vi "PeelDataCheck.vi"() -> ()   [LabVIEW 2012]
uses:
  <vilib>/addons/database/Connection.llb/DB Tools Open Connec (Path).vi
  <vilib>/addons/database/Connection.llb/Conn Execute.vi
  <vilib>/addons/database/Recordset.llb/Rec Fetch Recordset Data (R).vi
  <vilib>/addons/database/Recordset.llb/Rec Destroy - Connection.vi
  <vilib>/addons/database/_DB Variant To Data/Database Variant To Data.xnode
  <vilib>/addons/database/NI_Database_API.lvlib
  <vilib>/Utility/SMTP/NI_SMTPEmail.lvlib
panel:
  out "spreadsheet string":string
  out "array":string[][](array[string])
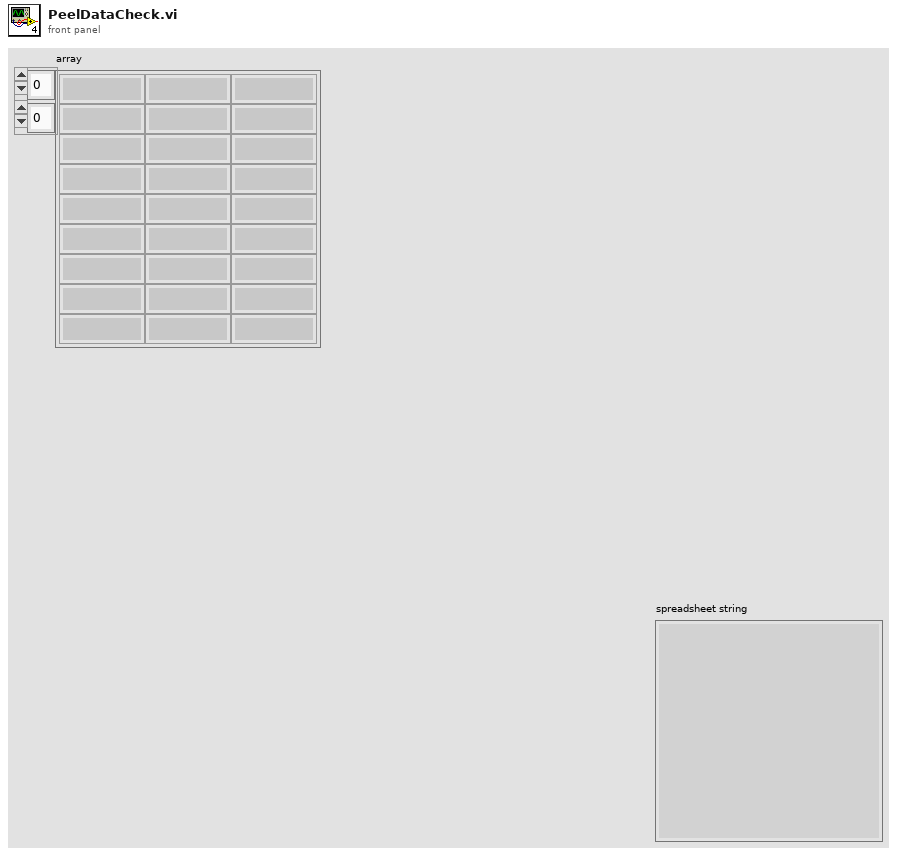
[diagram p1: front panel]
types:
  T1 = typedef "NI_Database_API.lvlib/Conn ObjectReference.ctl" = refnum<k1>
  T2 = typedef "NI_Database_API.lvlib/Rec ObjectReference.ctl" = refnum<k1>
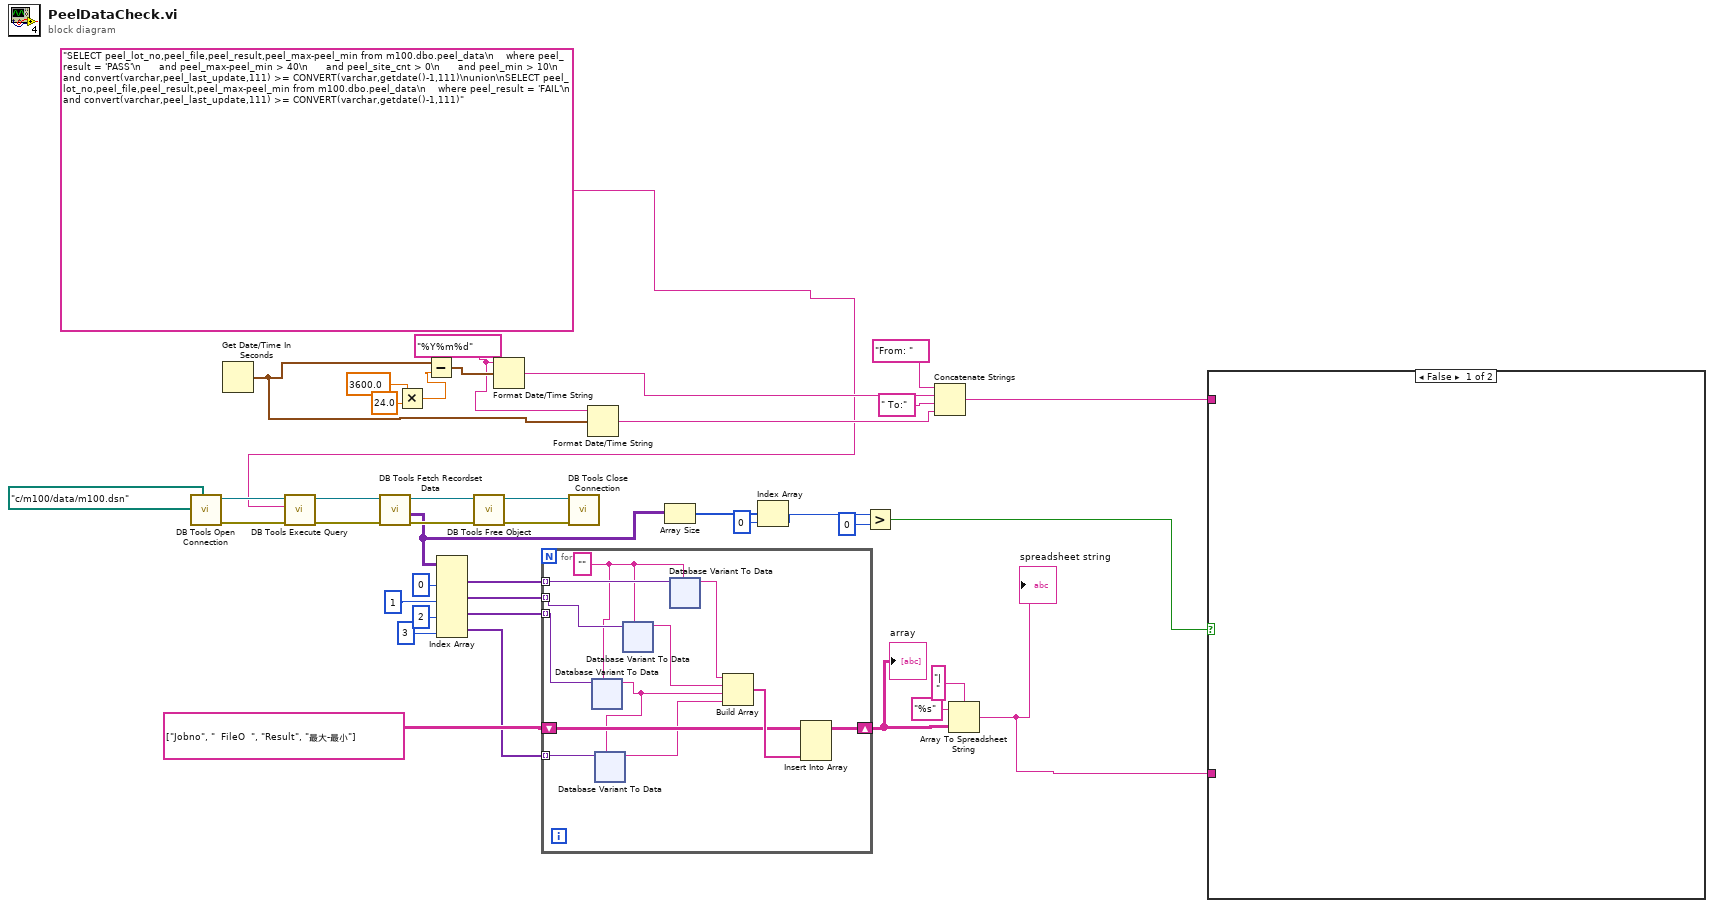
[diagram p0: block diagram]
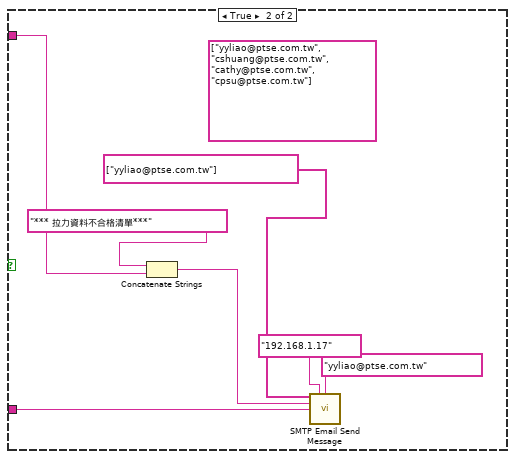
[diagram p2: hidden frame]
diagram:
  w16 = "%Y%m%d" ("time format string (%c)")
  n1 = call-poly <vilib>:"DB Tools Open Connection.vi"("connection information"=path "c:/m100/data/m100.dsn") -> ("error out"=w36:errorcluster, "connection reference"=w40:T1)  [unwired: 7 in]
  n2 = Get Date/Time In Seconds() -> (seconds since 1Jan1904=w17:timestamp)
  n3 = call-poly <vilib>:"DB Tools Execute Query.vi"("error in (no error)"=w36, "SQL query"="SELECT peel_lot_no,peel_file,peel_result,peel_max-peel_min from m100.dbo.peel_data\n    where peel_result = 'PASS'\n      and peel_max-peel_min > 40\n      and peel_site_cnt > 0\n      and peel_min > 10\n      and convert(varchar,peel_last_update,111) >= CONVERT(varchar,getdate()-1,111)\nunion\nSELECT peel_lot_no,peel_file,peel_result,peel_max-peel_min from m100.dbo.peel_data\n    where peel_result = 'FAIL'\n  and convert(varchar,peel_last_update,111) >= CONVERT(varchar,getdate()-1,111)", "connection reference"=w40) -> ("error out"=w35:errorcluster, "recordset reference"=w39:T2)  [unwired: 5 in]
  n4 = call-poly <vilib>:"DB Tools Fetch Recordset Data.vi"("error in (no error)"=w35, "recordset reference"=w39) -> ("error out"=w34:errorcluster, "recordset data"=w6:variant[][], "recordset reference out"=w38:T2)  [unwired: 3 in]
  n5 = Multiply(x=3600.0, y=24.0) -> (x*y=w20:dbl)
  n6 = Subtract(x=w17, y=w20) -> (x-y=w18:timestamp)
  n7 = Index Array(array=w6, index (col) #1=0 ("disabled index (col)"), index (col) #2=1 ("disabled index (row)"), index (col) #3=2 ("disabled index (col)"), index (col) #4=3 ("index (col)")) -> (element #1=w28:variant[], element #2=w27:variant[], element #3=w26:variant[], element #4=w8:variant[])  [unwired: 4 in]
  n8 = call-poly <vilib>:"DB Tools Free Object.vi"("error in (no error)"=w34, "recordset reference"=w38) -> ("error out"=w33:errorcluster, "connection reference"=w37:T1)  [unwired: 8 in]
  n9 = Format Date/Time String(time format string (%c)=w16, seconds (now)=w18) -> (date/time string=w14:string)  [unwired: 1 in]
  n10 = for {
    tunnel: w28 -> [w52] mode=indexing
    tunnel: w27 -> [w51] mode=indexing
    tunnel: w26 -> [w50] mode=indexing
    shift-right: [w45] -> w7
    shift-left: string[][] [["Jobno", "  FileO  ", "Result", "最大-最小"]] ("array") -> [w44]
    tunnel: w8 -> [w43] mode=indexing
    w49 = ""
    n11 = xnode "Database Variant To Data"("database variant"=w50, "type"=w49) -> ("data"=w42:string)  [unwired: 1 in, 1 out]
    n12 = xnode "Database Variant To Data"("database variant"=w43, "type"=w42) -> ("data"=w41:string)  [unwired: 1 in, 1 out]
    n13 = xnode "Database Variant To Data"("database variant"=w51, "type"=w49) -> ("data"=w47:string)  [unwired: 1 in, 1 out]
    n14 = xnode "Database Variant To Data"("database variant"=w52, "type"=w49) -> ("data"=w48:string)  [unwired: 1 in, 1 out]
    n15 = Build Array(w48, w47, w42, w41) -> (w46:string[])
    n16 = Insert Into Array(array=w44, new element=w46) -> (w45:string[][])  [unwired: 2 in]
  }
  "array" <- w7
  n17 = call <vilib>:"DB Tools Close Connection.vi"("error in (no error)"=w33, "connection reference"=w37) -> ()  [unwired: 5 in, 1 out]
  n18 = Format Date/Time String(time format string (%c)=w16, seconds (now)=w17) -> (date/time string=w12:string)  [unwired: 1 in]
  n19 = Array Size(array=w6) -> (size(s)=w5:i32[])
  n20 = Index Array(array=w5, index=0) -> (element=w3:i32)
  n21 = Greater?(x=w3, y=0) -> (0:w1:bool)
  n22 = Concatenate Strings("From: " ("string"), w14, " To:" ("string"), w12) -> (w11:string)
  n23 = Array To Spreadsheet String(delimiter (Tab)="| ", array=w7, 3:"%s" ("format string")) -> (spreadsheet string=w22:string)
  "spreadsheet string" <- w22
  n24 = case shown="False" w1 {
    tunnel: w22 -> [_ w185]
    tunnel: w11 -> [_ w182]
    frame False {
    }
    frame True {
      (unwired) string[] ["yyliao@ptse.com.tw", "cshuang@ptse.com.tw", "cathy@ptse.com.tw", "cpsu@ptse.com.tw"] ("recipients")
      n25 = Concatenate Strings("*** 拉力資料不合格清單***" ("subject ([No Subject])"), w182) -> (w184:string)
      n26 = call <vilib>:"SMTP Email Send Message.vi"("recipients"=string[] ["yyliao@ptse.com.tw"], "mail server"="192.168.1.17", "return address"="yyliao@ptse.com.tw", "subject ([No Subject])"=w184, "message"=w185) -> ()  [unwired: 9 in, 2 out]
    }
  }
